vi "STAGE+mono+counter_edit12.vi"() -> ()   [LabVIEW 2017]
uses:
  Control 1.ctl
panel:
  out "XY Graph":cluster{dbl[], dbl[]}(graph)
  out "Slide":u8(slide) max=10 step=10 scale=0.0..10.0
  out "?":cluster{dbl[], "Y":T1}(graph)
  in  "?":enum32{"DELAY", "COUNTER", "MONO", "PLOT"}(tab)
  out "Final time [ps]":dbl
  out "Current time [ps]":dbl
  out "Initial time [ps]":dbl
  in  "Set this as t0":bool
  in  "Axis":i32=1
  in  "Motor ON":bool
  in  "Motor OFF":bool
  out "Current Position [mm]":dbl
  out "Final Position [mm]":dbl
  in  "Data Points":i32=100
  out "Current Point":i32
  in  "Step Size [um]":i32=10
  in  "Target [mm]":dbl format="%.3f"
  in  "Move":bool
  out "Initial position [mm]":dbl
  in  "GPIB address":string="23"
  in  "Count Mode":u16(ring) items=["A,B for Preset T", "A-B for Preset T", "A+B for Preset T", "A for Preset B"]
  in  "Trigger mode":u16(ring) items=["10 MHz"=0, "Input 2"=2, "Input T"=3]
  in  "Channel A Input":u16(ring)=1 items=["10 MHz", "Input 1"]
  in  "Channel B Input":u16(ring)=2 items=["Input 1"=1, "Input 2"=2]
  in  "Number of Measurements\n to take at one point/ Number of Periods":u16=1 min=1 max=2000 step=1
  in  "Time between measurements\n at one point (s)/Dwell Time":dbl=0.002 min=0.002 max=60.0 step=0.001
  in  "gate A mode (CW:0)":i16(slide) scale=0.0..2.0 scale format="%.2f"
  out "Counts":i32
  in  "Integrating time, 10^-7 sec":dbl=10000000.0
  out "Mono port":T2(ring)
  out "Time delay":u32=450000 min=1
  out "Serial":u32=12345
  in  "Step size":dbl=10.0 min=0.0
  in  "Scan to":i32=4000
  in  "Scan from":i32=2600
  out "Current wavelength":dbl
  out "Grt#":u8=1 min=1 max=3 step=1
  in  "?":bool
  out "Groove/mm":u32=1200
  out "Blaze (nm)":u32=300
  in  "Array":dbl[](array[numeric])
  out "Timeout 2":bool
  in  "?":bool
  out "Timeout":bool
  in  "Collect Data!":bool
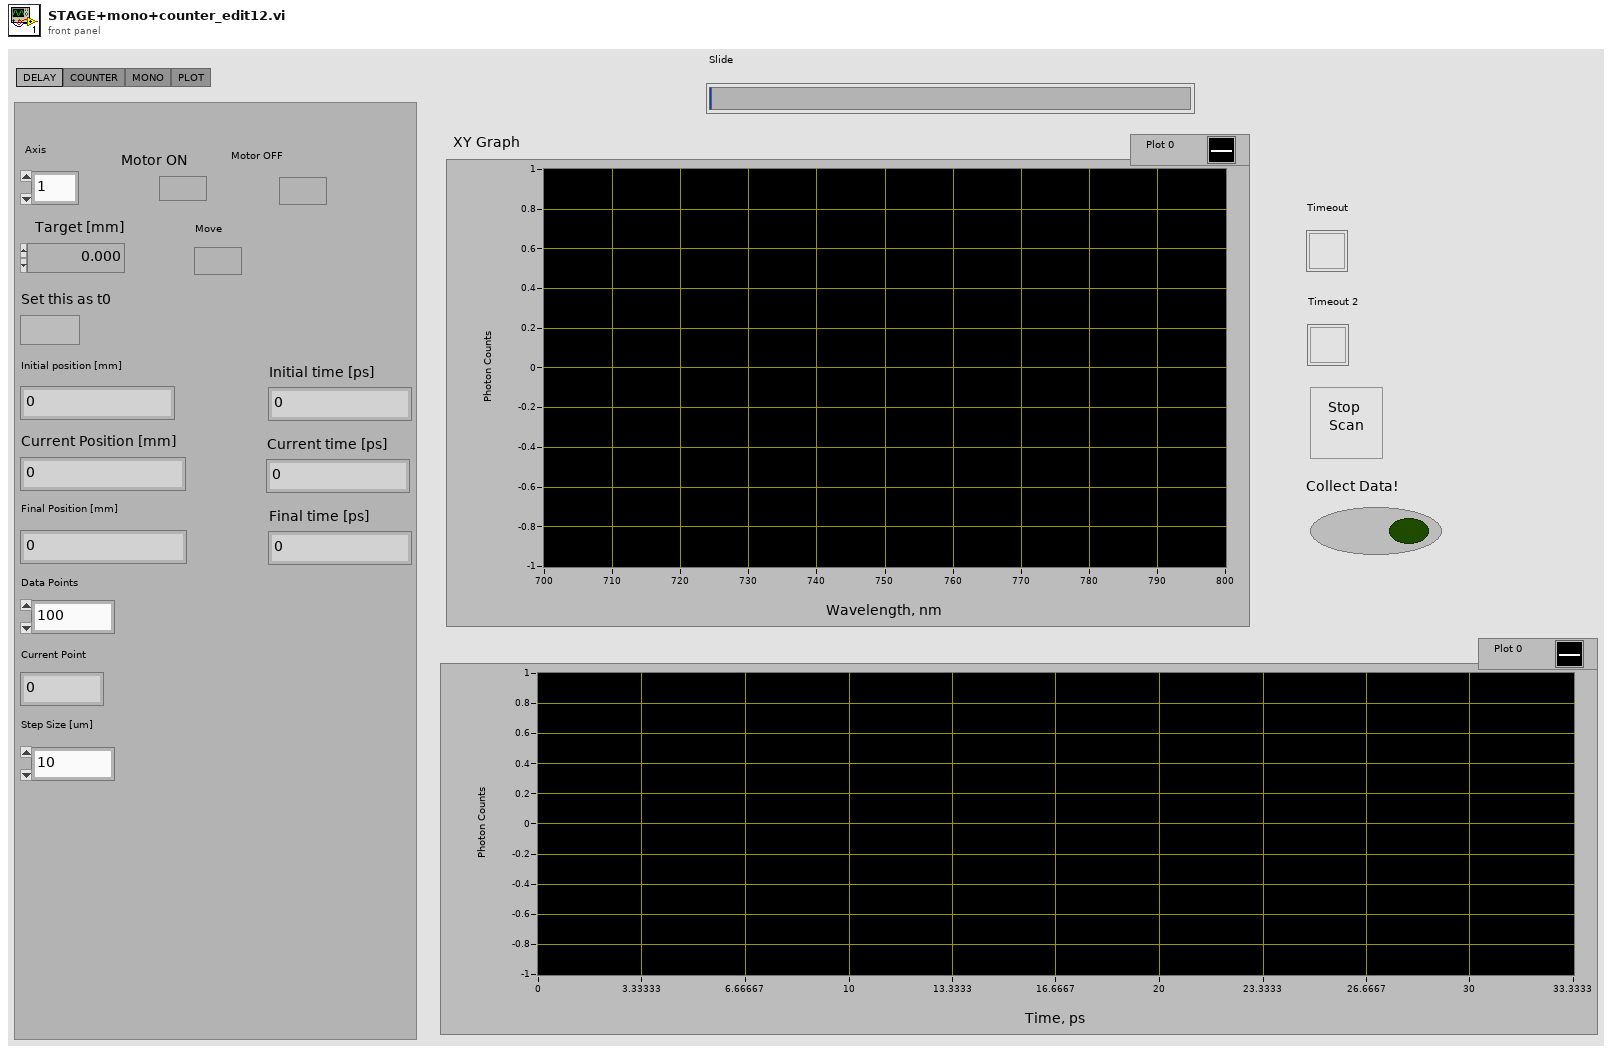
[diagram p1: front panel]
types:
  T1 = typedef "Control 1.ctl" = dbl[]
  T2 = enum8{"COM 1", "COM 2", "COM 3", "COM 4", "COM 5", "COM 6", "COM 7", "COM 8", "COM 9"}
  T3 = cluster{"input XON/XOFF":bool, "input HW Handshake":bool, "input alt HW HShk":bool, "output XON/XOFF":bool, "output HW Handshake":bool, "output alt HW HShk":bool, "XOFF byte":u8, "XON byte":u8, "parity error byte":u16}
  T4 = enum16{"no parity", "odd parity", "even parity", "mark parity", "space parity"}
  T5 = cluster{"Y[0]":dbl, "Y[1]":dbl, "Y[2]":dbl, "Y[3]":dbl, "Y[4]":dbl, "Y[5]":dbl, "Y[6]":dbl, "Y[7]":dbl, "Y[8]":dbl}
  T6 = typedef "NI_Matrix.lvlib/RealMatrix.ctl" = dbl[][]
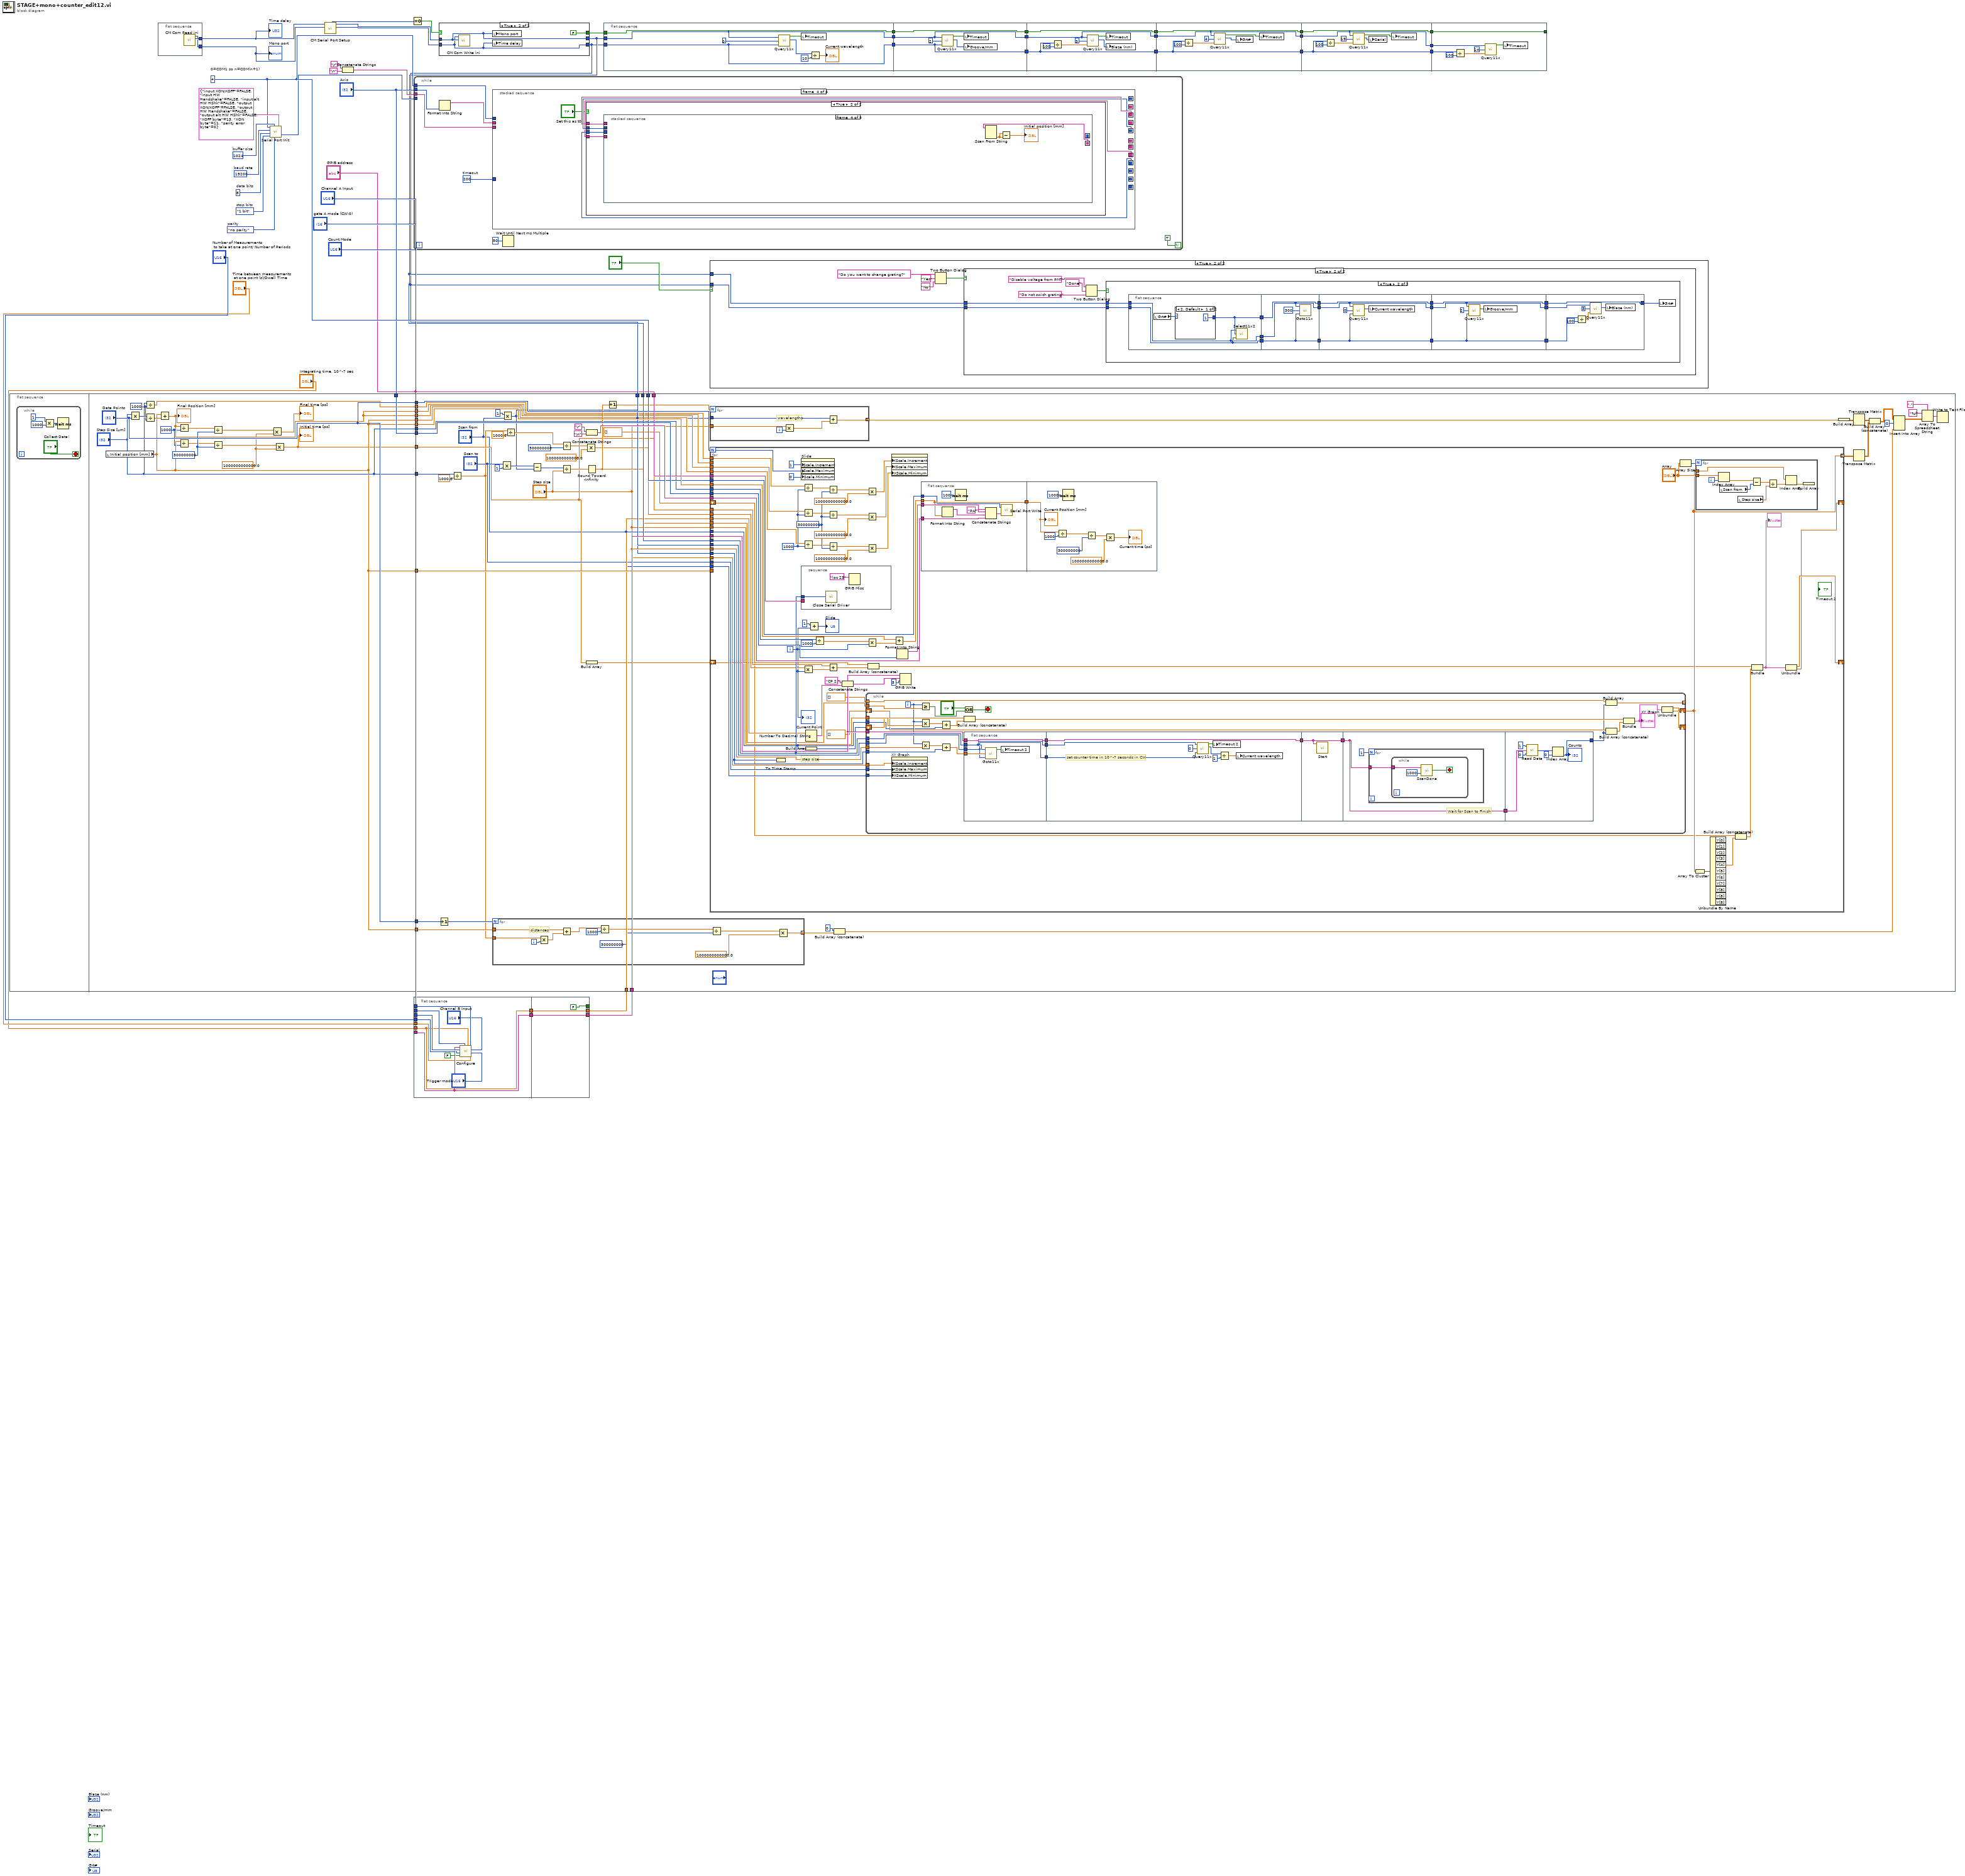
[diagram p0: block diagram]
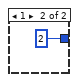
[diagram p5: hidden frame]
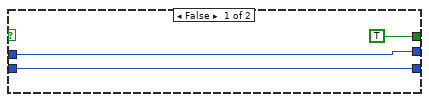
[diagram p6: hidden frame]
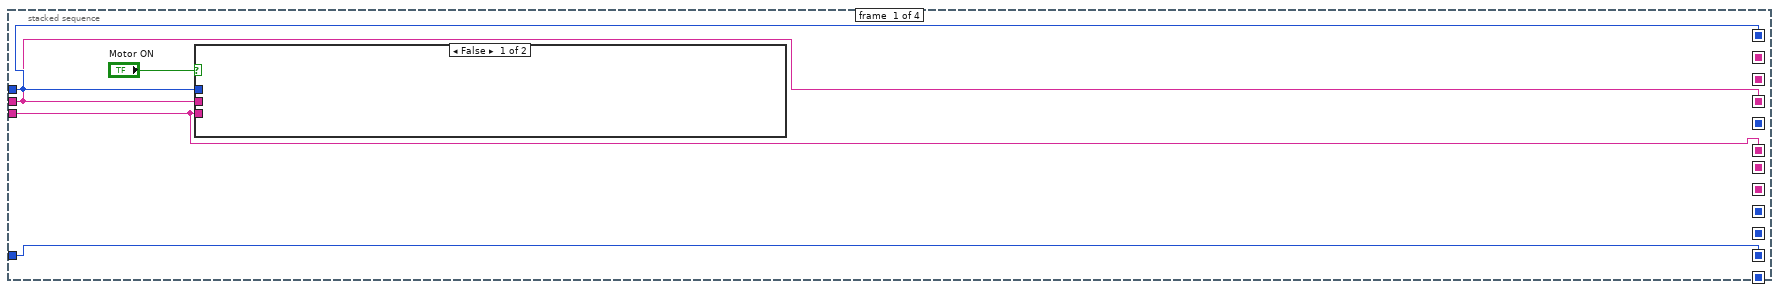
[diagram p7: hidden frame]
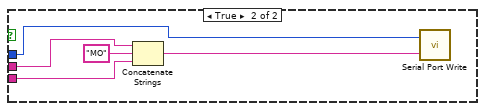
[diagram p8: hidden frame]
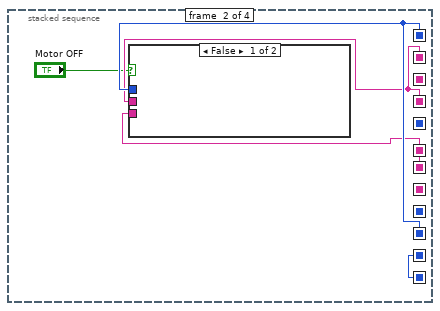
[diagram p9: hidden frame]
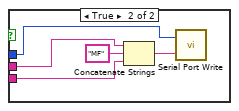
[diagram p10: hidden frame]
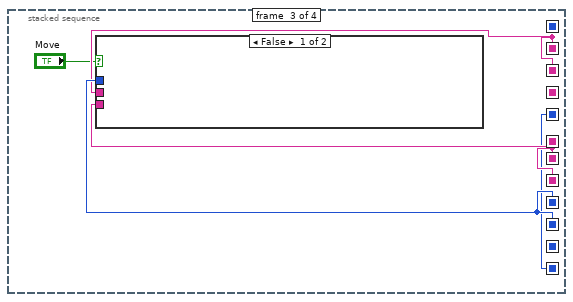
[diagram p11: hidden frame]
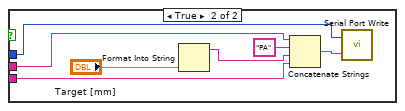
[diagram p12: hidden frame]
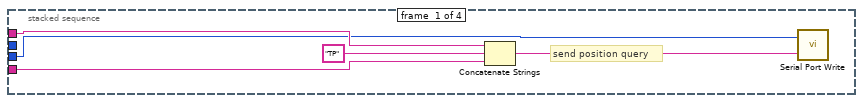
[diagram p14: hidden frame]
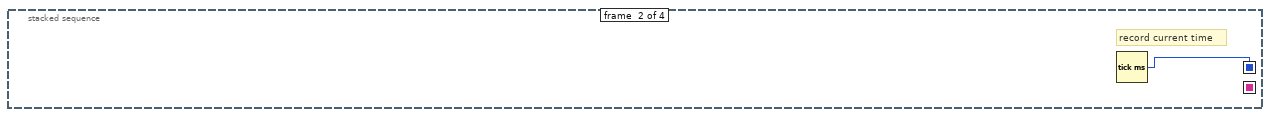
[diagram p15: hidden frame]
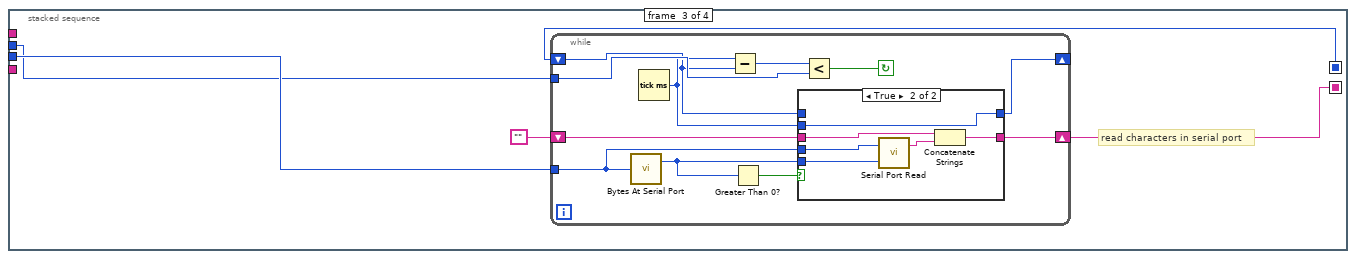
[diagram p16: hidden frame]
diagram:
  w55 = u32 19200  # baud rate
  w54 = u16 8  # data bits
  w53 = enum16{"1 bit", "1.5 bits", "2 bits"}."1 bit"  # stop bits
  w57 = T4."no parity"  # parity
  w52 = 4  # 0=COM1 so n=COM(n+1)
  w56 = u16 1024  # buffer size
  n1 = flat-sequence {
    tunnel: ["Data Points"] -> w61
    tunnel: "Axis" -> [w83]
    tunnel: [w75] -> w60
    tunnel: [w83] -> w59
    tunnel: ["Step Size [um]"] -> w12
    tunnel: [w75] -> w11
    tunnel: ["Step Size [um]"] -> w10
    tunnel: ["Data Points"] -> w9
    tunnel: [w75] -> w8
    tunnel: [w74] -> w7
    tunnel: [w75] -> w4
    tunnel: [w74] -> w3
    tunnel: [w77] -> w2
    tunnel: [w66] -> w1
    tunnel: w61 -> [w141]
    tunnel: w60 -> [w140]
    tunnel: w59 -> [w139]
    tunnel: w52 -> [w135]
    tunnel: w16 -> [w134]
    tunnel: w15 -> [w133]
    tunnel: w14 -> [w132]
    tunnel: "GPIB address" -> [w131]
    tunnel: w12 -> [w118]
    tunnel: w11 -> [w116]
    tunnel: w10 -> [w115]
    tunnel: w9 -> [w113]
    tunnel: w8 -> [w106]
    tunnel: w7 -> [w105]
    tunnel: w6 -> [w104]
    tunnel: w4 -> [w102]
    tunnel: w3 -> [w101]
    tunnel: w2 -> [w100]
    tunnel: w1 -> [w96]
    frame #0 {
      n2 = while {
        stop <- "Collect Data!" stop-if-true
        n3 = Multiply(x=1, y=1000) -> (x*y=w65:i32)
        n4 = Wait (ms)(milliseconds to wait=w65) -> ()  [unwired: 1 out]
      }
    }
    frame #1 {
      w67 = 1000000000000.0
      w73 = 1000
      w76 = 300000000
      w78 = 1000
      n5 = local read "Initial position [mm]"() -> (w75:dbl)
      n6 = Multiply(x="Step Size [um]", y="Data Points") -> (x*y=w82:i32)
      n7 = Divide(x="Step Size [um]", y=w78) -> (x/y=w77:dbl)
      n8 = Divide(x=w82, y=w78) -> (x/y=w81:dbl)
      n9 = Add(x=w75, y=w81) -> (x+y=w74:dbl)
      "Final Position [mm]" <- w74
      n10 = Divide(x=w74, y=w73) -> (x/y=w72:dbl)
      n11 = Divide(x=w75, y=w73) -> (x/y=w71:dbl)
      n12 = Divide(x=w72, y=w76) -> (x/y=w69:dbl)
      n13 = Divide(x=w71, y=w76) -> (x/y=w70:dbl)
      n14 = Multiply(x=w69, y=w67) -> (x*y=→"Final time [ps]":dbl)
      n15 = Multiply(x=w70, y=w67) -> (x*y=w66:dbl)
      "Initial time [ps]" <- w66
    }
    frame #2 {
      n16 = Increment(x=w113) -> (x+1=w114:i32)
      n17 = Divide(x=w118, y=1000.0) -> (x/y=w90:dbl)
      n18 = for {
        N: w114 -> [_]
        tunnel: w90 -> [w152]
        tunnel: w116 -> [w150]
        tunnel: [w143] -> w112 mode=indexing
        i -> [w151]
        # "distances"
        n19 = Multiply(x=w152, y=w151) -> (x*y=w149:dbl)
        n20 = Add(x=w150, y=w149) -> (x+y=w148:dbl)
        n21 = Divide(x=w148, y=1000) -> (x/y=w142:dbl)
        n22 = Divide(x=w142, y=300000000) -> (x/y=w145:dbl)
        n23 = Multiply(x=w145, y=1000000000000.0) -> (x*y=w143:dbl)
      }
      n24 = Multiply(x="Scan to", y=1) -> (x*y=w97:i32)
      n25 = Multiply(x=1, y="Scan from") -> (x*y=w86:i32)
      n26 = Divide(x=w90, y=1000.0) -> (x/y=w91:dbl)
      n27 = Subtract(x=w97, y=w86) -> (x-y=w126:i32)
      n28 = Divide(x=w91, y=300000000) -> (x/y=w93:dbl)
      n29 = Divide(x=w126, y="Step size") -> (x/y=w125:dbl)
      n30 = Multiply(x=w93, y=1000000000000.0) -> (x*y=w89:dbl)
      n31 = Concatenate Strings("\r", "\n") -> (w136:string)
      n32 = Round Toward -Infinity(1:w125) -> (0:w124:dbl)
      n33 = Build Array(w96) -> (w98:dbl[])
      n34 = Increment(x=w124) -> (x+1=w85:dbl)
      n35 = for {
        N: w85 -> [_]
        tunnel: "Step size" -> [w157]
        tunnel: w86 -> [w155]
        tunnel: [w153] -> w84 mode=indexing
        i -> [w156]
        # "wavelengths"
        n36 = Multiply(x=w157, y=w156) -> (x*y=w154:dbl)
        n37 = Add(x=w155, y=w154) -> (x+y=w153:dbl)
      }
      n38 = for {
        N: w141 -> [w193]
        tunnel: w140 -> [w227]
        tunnel: w115 -> [w223]
        tunnel: w139 -> [w220]
        tunnel: w136 -> [w217]
        tunnel: w135 -> [w218]
        tunnel: w134 -> [w216]
        tunnel: w133 -> [w213]
        tunnel: w132 -> [w215]
        tunnel: w131 -> [w214]
        tunnel: [w160] -> w121 mode=indexing
        tunnel: w86 -> [w208]
        tunnel: "Step size" -> [w207]
        tunnel: w124 -> [w206]
        tunnel: w106 -> [_]
        tunnel: w105 -> [_]
        tunnel: w104 -> [w204]
        tunnel: "Scan to" -> [w203]
        tunnel: "Scan from" -> [w202]
        tunnel: "Step size" -> [w164]
        tunnel: w102 -> [w188]
        tunnel: w101 -> [w186]
        tunnel: w100 -> [w189]
        tunnel: w89 -> [w173]
        shift-right: [w200] -> _
        shift-left: w98 -> [w167]
        shift-right: [w197] -> _
        shift-left: T1 [] ("Y") -> [w158]
        tunnel: w96 -> [w196]
        tunnel: "Scan from" -> [w165]
        tunnel: "Step size" -> [w166]
        i -> [w172]
        w187 = 1000
        w190 = 300000000
        # "step size"
        n39 = To Time Stamp(1:w208) -> ()  [unwired: 1 out]
        n40 = property on="Slide" class="Slide (strict)"("Scale.Increment"=1, "Scale.Maximum"=w193, "Scale.Minimum"=0) -> ()  [unwired: 2 in, 2 out]
        n41 = stacked-sequence {
          tunnel: w213 -> [w299]
          tunnel: w214 -> [_]
          frame #0 {
            n42 = call <vilib>:"Close Serial Driver.vi"("port number"=w299) -> ()  [unwired: 1 out]
            n43 = GPIB Misc(0:"loc 23" ("command string")) -> ()  [unwired: 1 in, 3 out]
          }
        }
        n44 = Divide(x=w189, y=w187) -> (x/y=w185:dbl)
        n45 = Divide(x=w186, y=w187) -> (x/y=w183:dbl)
        n46 = Divide(x=w188, y=w187) -> (x/y=w184:dbl)
        n47 = Multiply(x=w173, y=w172) -> (x*y=w201:dbl)
        n48 = Number To Decimal String(number=w204) -> (decimal integer string=w211:string)  [unwired: 1 in]
        n49 = Build Array(w165) -> (w169:i32[])
        n50 = Add(x=1, y=w172) -> (x+y=→"Slide":i32)
        n51 = Divide(x=w223, y=1000) -> (x/y=w222:dbl)
        n52 = Divide(x=w185, y=w190) -> (x/y=w179:dbl)
        n53 = Divide(x=w183, y=w190) -> (x/y=w175:dbl)
        n54 = Divide(x=w184, y=w190) -> (x/y=w177:dbl)
        n55 = Add(x=w196, y=w201) -> (x+y=w195:dbl)
        n56 = Concatenate Strings("CP 2,", w211) -> (w209:string)
        n57 = while {
          tunnel: w213 -> [w270]
          tunnel: w215 -> [w269]
          tunnel: w216 -> [w265]
          tunnel: w208 -> [w257]
          tunnel: w207 -> [w256]
          tunnel: w206 -> [w255]
          tunnel: w203 -> [w242]
          tunnel: w202 -> [w241]
          tunnel: w164 -> [w240]
          tunnel: w166 -> [w253]
          shift-right: [w248] -> w160
          shift-left: dbl[] [] ("Y") -> [w247]
          shift-right: [w237] -> _
          shift-left: w169 -> [w251]
          tunnel: w165 -> [w245]
          tunnel: dbl[] [] ("Y") -> [w238] mode=indexing
          tunnel: [w239] -> _ mode=indexing
          i -> [w254]
          stop <- w268 stop-if-true
          n58 = property on="XY Graph" class="XYGraph (strict)"("XScale.Increment"=w240, "XScale.Maximum"=w242, "XScale.Minimum"=w241) -> ()  [unwired: 2 in, 2 out]
          n59 = Greater Or Equal?(x=w254, y=w255) -> (x >= y?=w266:bool)
          n60 = Multiply(x=w254, y=w253) -> (x*y=w252:dbl)
          n61 = Multiply(x=w254, y=w256) -> (x*y=w271:dbl)
          n62 = Add(x=w252, y=w245) -> (x+y=w250:dbl)
          n63 = Add(x=w271, y=w257) -> (x+y=w258:dbl)
          n64 = Or(x="?", y=w266) -> (x .or. y?=w268:bool)
          n65 = Build Array (concatenate)(w251, w250) -> (w249:dbl[])
          n66 = flat-sequence {
            tunnel: w258 -> [w276]
            tunnel: w270 -> [w275]
            tunnel: [w275] -> w264
            tunnel: w269 -> [w274]
            tunnel: [w274] -> w263
            tunnel: w265 -> [w272]
            tunnel: [w272] -> w262
            tunnel: w264 -> [w283]
            tunnel: w263 -> [w282]
            tunnel: w262 -> [w280]
            tunnel: [w280] -> w261
            tunnel: w261 -> [w285]
            tunnel: [w285] -> w260
            tunnel: w260 -> [w286]
            tunnel: [w286] -> w259
            tunnel: w259 -> [w293]
            tunnel: [w292] -> w244
            frame #0 {
              n67 = call "Goto11x.vi"("time delay"=w274, "WAVELENGTH"=w276, "port number"=w275) -> ("timeout"=w273:bool)  [unwired: 2 out]
              n68 = local write "Timeout 2"(w273) -> ()
            }
            frame #1 {
              # "set counter time in 10^-7 seconds in CW"
              n69 = call "Query11x.vi"("port number"=w283, "QUERY"=0, "time delay"=w282) -> ("timeout"=w281:bool, "STATUS MESSAGE"=w279:u16)  [unwired: 2 out]
              n70 = local write "Timeout 2"(w281) -> ()
              n71 = Divide(x=w279, y=1) -> (x/y=w278:dbl)
              n72 = local write "Current wavelength"(w278) -> ()
            }
            frame #2 {
              n73 = call "Start.vi"("GPIB Address"=w285) -> ()  [unwired: 9 in]
            }
            frame #3 {
              # "Wait for Scan to Finish"
              n74 = for {
                N: 1 -> [_]
                tunnel: w286 -> [w288]
                n75 = while {
                  tunnel: w288 -> [w289]
                  stop <- w291 stop-if-true
                  n76 = call "ScanDone.vi"("Wait (ms)"=1000, "GPIB Address"=w289) -> ("Scan Finished?"=w291:bool)
                }
              }
            }
            frame #4 {
              n77 = call "Read Data.vi"("Channel Number"=0, "GPIB Address"=w293, "Number of Datapoints"=1) -> ("Data"=w294:i32[])
              n78 = Index Array(array=w294, index=0) -> (element=w292:i32)
              "Counts" <- w292
            }
          }
          n79 = Build Array(w238, w244) -> (w239:dbl[])
          n80 = Build Array (concatenate)(w247, w244) -> (w246:dbl[])
          n81 = Bundle(w249, w246) -> (w243:cluster{dbl[], dbl[]})  [unwired: 1 in]
          "XY Graph" <- w243
          n82 = Unbundle(w243) -> (w237:dbl[], w248:dbl[])
        }
        n83 = Multiply(x=w179, y=1000000000000.0) -> (x*y=w178:dbl)
        n84 = Multiply(x=w175, y=1000000000000.0) -> (x*y=w174:dbl)
        n85 = Multiply(x=w177, y=1000000000000.0) -> (x*y=w176:dbl)
        n86 = Multiply(x=w222, y=w172) -> (x*y=w226:dbl)
        n87 = Build Array (concatenate)(w167, w195) -> (w159:dbl[])
        n88 = property class="XYGraph (strict)"("XScale.Increment"=w178, "XScale.Maximum"=w174, "XScale.Minimum"=w176) -> ()  [unwired: 2 in, 2 out]
        n89 = Add(x=w227, y=w226) -> (x+y=w225:dbl)
        n90 = Format Into String(w220) -> (resulting string=w219:string)  [unwired: 3 in, 1 out]
        n91 = GPIB Write(0:w216, 1:w209, 2:i16 5 ("mode (0)")) -> ()  [unwired: 2 in, 2 out]
        n92 = flat-sequence {
          tunnel: w225 -> [w302]
          tunnel: [w302] -> w221
          tunnel: w217 -> [w304]
          tunnel: w219 -> [w303]
          tunnel: w218 -> [w300]
          tunnel: w221 -> [w313]
          frame #0 {
            n93 = Format Into String(w302) -> (resulting string=w301:string)  [unwired: 3 in, 1 out]
            n94 = Wait (ms)(milliseconds to wait=u32 100) -> ()  [unwired: 1 out]
            n95 = Concatenate Strings(w303, "PA" ("Substring"), w301, w304) -> (w306:string)
            n96 = call <vilib>:"Serial Port Write.vi"("string to write"=w306, "port number"=w300) -> ()  [unwired: 1 out]
          }
          frame #1 {
            n97 = Divide(x=w313, y=1000) -> (x/y=w311:dbl)
            n98 = Wait (ms)(milliseconds to wait=u32 1000) -> ()  [unwired: 1 out]
            n99 = Divide(x=w311, y=300000000) -> (x/y=w310:dbl)
            n100 = Multiply(x=w310, y=1000000000000.0) -> (x*y=→"Current time [ps]":dbl)
            "Current Position [mm]" <- w313
          }
        }
        n101 = Array Size(array="Array") -> (size(s)=w162:i32)
        n102 = Array To Cluster(array=w160) -> (cluster=w205:T5)
        n103 = for {
          N: w162 -> [_]
          tunnel: "Array" -> [w236]
          tunnel: w160 -> [w230]
          i -> [w235]
          n104 = Index Array(array=w236, index=w235) -> (element=w234:dbl)
          n105 = local read "Scan from"() -> (w233:i32)
          n106 = local read "Step size"() -> (w231:dbl)
          n107 = Subtract(x=w234, y=w233) -> (x-y=w232:dbl)
          n108 = Divide(x=w232, y=w231) -> (x/y=w229:dbl)
          n109 = Index Array(array=w230, index=w229) -> (element=w228:dbl)
          n110 = Build Array(w228) -> ()  [unwired: 1 out]
        }
        n111 = Unbundle By Name(w205) -> ("Y[4]"=w199:dbl)  [unwired: 10 out]
        n112 = Build Array (concatenate)(w158, w199) -> (w198:T1)
        n113 = Bundle(w159, "Y"=w198) -> (w194:cluster{dbl[], "Y":T1})  [unwired: 1 in]
        "?" <- w194
        n114 = Unbundle(w194) -> (w200:dbl[], "Y"=w197:T1)
        "Current Point" <- w172
      }
      n115 = Build Array (concatenate)(0, w112) -> (w109:dbl[])
      n116 = Build Array(w84) -> (w122:dbl[][])
      n117 = Transpose Matrix(1:w122) -> (0:w120:dbl[][])
      n118 = Transpose Matrix(1:w121) -> (0:w119:dbl[][])
      n119 = Build Array (concatenate)(w120, w119) -> (w108:T6)
      n120 = Insert Into Array(array=w108, index (row)=0, new element=w109) -> (w107:T6)  [unwired: 1 in]
      n121 = Array To Spreadsheet String(delimiter (Tab)=",", array=w107, 3:"%f" ("format string")) -> (spreadsheet string=w123:string)
      n122 = Write to Text File(text=w123) -> ()  [unwired: 3 in, 3 out]
    }
  }
  n123 = flat-sequence {
    tunnel: [w317] -> w30
    tunnel: [w316] -> w29
    frame #0 {
      n124 = call "CM Com Read ini.vi"() -> ("Mono port"=w316:T2, "time delay1"=w317:u32)  [unwired: 7 in]
    }
  }
  n125 = call <vilib>:"Serial Port Init.vi"("flow control etc."=T3 {"input XON/XOFF"=FALSE, "input HW Handshake"=FALSE, "input alt HW HShk"=FALSE, "output XON/XOFF"=FALSE, "output HW Handshake"=FALSE, "output alt HW HShk"=FALSE, "XOFF byte"=13, "XON byte"=11, "parity error byte"=0}, "parity"=w57, "buffer size"=w56, "stop bits"=w53, "data bits"=w54, "baud rate"=w55, "port number"=w52) -> ("error code"=w51:i32)
  n126 = call "CM Serial Port Setup.vi"("COM port"=w29, "time delay"=w30) -> ("time delay1"=w25:u32, "DK port Out"=w26:T2, "error code"=w28:i32)  [unwired: 7 in]
  n127 = Concatenate Strings("\r", "\n") -> (w47:string)
  n128 = Equal To 0?(x=w28) -> (x = 0?=w27:bool)
  n129 = while {
    tunnel: w52 -> [w320]
    tunnel: w47 -> [w321]
    tunnel: w51 -> [_]
    tunnel: "Axis" -> [w318]
    stop <- TRUE continue-if-true
    w319 = u32 200  # timeout
    n130 = Format Into String(w318) -> (resulting string=w322:string)  [unwired: 3 in, 1 out]
    n131 = stacked-sequence {
      seq-local: [w327 _ _ _] -> [_ w338 _ _]
      seq-local: [w326 _ _ _] -> [_ w337 _ _]
      seq-local: [w328 _ _ _] -> [_ w339 _ _]
      seq-local: [w325 _ _ _] -> [_ w335 _ _]
      seq-local: [_ w338 _ _] -> [_ _ w348 _]
      seq-local: [_ w337 _ _] -> [_ _ w347 _]
      seq-local: [_ w339 _ _] -> [_ _ w349 _]
      seq-local: [_ w335 _ _] -> [_ _ w345 _]
      seq-local: [_ _ w348 _] -> [_ _ _ w361]
      seq-local: [_ _ w347 _] -> [_ _ _ w358]
      seq-local: [_ _ w349 _] -> [_ _ _ w360]
      seq-local: [_ _ w345 _] -> [_ _ _ w359]
      tunnel: w322 -> [w327 _ _ _]
      tunnel: w321 -> [w326 _ _ _]
      tunnel: w320 -> [w328 _ _ _]
      tunnel: w319 -> [w325 _ _ _]
      frame #0 {
        n132 = case shown="False" "Motor ON" {
          tunnel: w328 -> [_ w334]
          tunnel: w327 -> [_ w331]
          tunnel: w326 -> [_ w330]
          frame False {
          }
          frame True {
            n133 = Concatenate Strings(w331, "MO" ("Substring"), w330) -> (w332:string)
            n134 = call <vilib>:"Serial Port Write.vi"("string to write"=w332, "port number"=w334) -> ()  [unwired: 1 out]
          }
        }
      }
      frame #1 {
        n135 = case shown="False" "Motor OFF" {
          tunnel: w339 -> [_ w344]
          tunnel: w338 -> [_ w341]
          tunnel: w337 -> [_ w340]
          frame False {
          }
          frame True {
            n136 = Concatenate Strings(w341, "MF" ("Substring"), w340) -> (w342:string)
            n137 = call <vilib>:"Serial Port Write.vi"("string to write"=w342, "port number"=w344) -> ()  [unwired: 1 out]
          }
        }
      }
      frame #2 {
        n138 = case shown="False" "Move" {
          tunnel: w349 -> [_ w356]
          tunnel: w348 -> [_ w353]
          tunnel: w347 -> [_ w352]
          frame False {
          }
          frame True {
            n139 = Format Into String("Target [mm]") -> (resulting string=w350:string)  [unwired: 3 in, 1 out]
            n140 = Concatenate Strings(w353, "PA" ("Substring"), w350, w352) -> (w354:string)
            n141 = call <vilib>:"Serial Port Write.vi"("string to write"=w354, "port number"=w356) -> ()  [unwired: 1 out]
          }
        }
      }
      frame #3 {
        n142 = case shown="True" "Set this as t0" {
          tunnel: w361 -> [_ w365]
          tunnel: w360 -> [_ w364]
          tunnel: w359 -> [_ w363]
          tunnel: w358 -> [_ w362]
          frame False {
          }
          frame True {
            n143 = stacked-sequence {
              seq-local: [_ w371 _ _] -> [_ _ w373 _]
              seq-local: [_ _ w372 _] -> [_ _ _ w398]
              tunnel: w365 -> [w368 _ _ _]
              tunnel: w364 -> [w367 _ w376 _]
              tunnel: w363 -> [_ _ w374 _]
              tunnel: w362 -> [w366 _ _ _]
              frame #0 {
                # "send position query"
                n144 = Concatenate Strings(w368, "TP" ("Substring"), w366) -> (w369:string)
                n145 = call <vilib>:"Serial Port Write.vi"("string to write"=w369, "port number"=w367) -> ()  [unwired: 1 out]
              }
              frame #1 {
                # "record current time"
                n146 = Tick Count (ms)() -> (millisecond timer value=w371:u32)
              }
              frame #2 {
                # "read characters in serial port"
                n147 = while {
                  shift-left: w373 -> [w377]
                  shift-right: [w378] -> _
                  tunnel: w374 -> [w381]
                  shift-left: "" -> [w384]
                  shift-right: [w383] -> w372
                  tunnel: w376 -> [w385]
                  stop <- w380 continue-if-true
                  n148 = call <vilib>:"Bytes At Serial Port.vi"("port number"=w385) -> ("byte count"=w386:u32)  [unwired: 1 out]
                  n149 = Tick Count (ms)() -> (millisecond timer value=w379:u32)
                  n150 = Subtract(x=w379, y=w377) -> (x-y=w382:u32)
                  n151 = Greater Than 0?(x=w386) -> (x > 0?=w387:bool)
                  n152 = case shown="True" w387 {
                    tunnel: w386 -> [_ w395]
                    tunnel: w385 -> [_ w394]
                    tunnel: w384 -> [w389 w392]
                    tunnel: [w389 w391] -> w383
                    tunnel: [w388 w390] -> w378
                    tunnel: w379 -> [_ w390]
                    tunnel: w377 -> [w388 _]
                    frame False {
                    }
                    frame True {
                      n153 = call <vilib>:"Serial Port Read.vi"("requested byte count"=w395, "port number"=w394) -> ("string read"=w393:string)  [unwired: 1 out]
                      n154 = Concatenate Strings(w392, w393) -> (w391:string)
                    }
                  }
                  n155 = Less?(x=w382, y=w381) -> (x < y?=w380:bool)
                }
              }
              frame #3 {
                n156 = Scan From String(input string=w398) -> (output 1=w396:dbl)  [unwired: 4 in, 3 out]
                n157 = Subtract(x=w396, y=w396) -> (x-y=→"Initial position [mm]":dbl)
              }
            }
          }
        }
      }
    }
    n158 = Wait Until Next ms Multiple(millisecond multiple=u32 50) -> ()  [unwired: 1 out]
  }
  n159 = flat-sequence {
    tunnel: "GPIB address" -> [w406]
    tunnel: [w406] -> w31
    tunnel: "Count Mode" -> [w407]
    tunnel: "Number of Measurements\n to take at one point/ Number of Periods" -> [w404]
    tunnel: "Time between measurements\n at one point (s)/Dwell Time" -> [w403]
    tunnel: "Channel A Input" -> [w408]
    tunnel: "gate A mode (CW:0)" -> [w400]
    tunnel: "Integrating time, 10^-7 sec" -> [w399]
    tunnel: [w399] -> w5
    tunnel: w31 -> [w410]
    tunnel: [w410] -> w16
    tunnel: [FALSE] -> _
    tunnel: [w409] -> w6
    tunnel: w5 -> [w409]
    frame #0 {
      n160 = call "Configure.vi"("Dwell Time (s)"=w403, "Channel T Input"="Trigger mode", "Channel B Input"="Channel B Input", "Channel A Input"=w408, "Integrating time, 10^-7 sec"=w399, "gate mode (CW:0)"=w400, "Scan End Mode"=FALSE, "Number of Periods"=w404, "Count Mode"=w407, "GPIB Address"=w406) -> ()
    }
    frame #1 {
    }
  }
  n161 = case shown="True" w27 {
    tunnel: w26 -> [w414 w417]
    tunnel: w25 -> [w413 w416]
    tunnel: [w414 w417] -> w15
    tunnel: [w413 w416] -> w14
    tunnel: [TRUE FALSE] -> w24
    frame False {
    }
    frame True {
      n162 = call "CM Com Write ini.vi"("time delay1"=w417, "Mono port"=w416) -> ()  [unwired: 7 in]
      n163 = local write "Mono port"(w417) -> ()
      n164 = local write "Time delay"(w416) -> ()
    }
  }
  n165 = flat-sequence {
    tunnel: w14 -> [w423]
    tunnel: [w423] -> w46
    tunnel: w15 -> [w425]
    tunnel: [w425] -> w45
    tunnel: w24 -> [w421]
    tunnel: [w421] -> w44
    tunnel: w46 -> [w428]
    tunnel: [w428] -> w43
    tunnel: w45 -> [w430]
    tunnel: [w430] -> w42
    tunnel: w44 -> [w426]
    tunnel: [w426] -> w41
    tunnel: w43 -> [w438]
    tunnel: [w438] -> w40
    tunnel: w42 -> [w435]
    tunnel: [w435] -> w39
    tunnel: w41 -> [w432]
    tunnel: [w432] -> w38
    tunnel: w40 -> [w446]
    tunnel: [w446] -> w37
    tunnel: w39 -> [w443]
    tunnel: [w443] -> w36
    tunnel: w38 -> [w440]
    tunnel: [w440] -> w35
    tunnel: w37 -> [w454]
    tunnel: [w454] -> w34
    tunnel: w36 -> [w451]
    tunnel: [w451] -> w33
    tunnel: w35 -> [w448]
    tunnel: [w448] -> w32
    tunnel: w34 -> [w461]
    tunnel: w33 -> [w458]
    tunnel: [w456] -> _
    tunnel: w32 -> [w456]
    frame #0 {
      n166 = call "Query11x.vi"("port number"=w425, "QUERY"=u16 0, "time delay"=w423) -> ("timeout"=w422:bool, "STATUS MESSAGE"=w420:u16)  [unwired: 2 out]
      n167 = local write "Timeout"(w422) -> ()
      n168 = Divide(x=w420, y=10 ("Numeric")) -> (x/y=→"Current wavelength":dbl)
    }
    frame #1 {
      n169 = call "Query11x.vi"("port number"=w430, "QUERY"=u16 2, "time delay"=w428) -> ("timeout"=w427:bool, "STATUS MESSAGE"=w429:u16)  [unwired: 2 out]
      n170 = local write "Timeout"(w427) -> ()
      n171 = local write "Groove/mm"(w429) -> ()
    }
    frame #2 {
      n172 = Divide(x=w438, y=i16 100 ("device (1)")) -> (x/y=w436:dbl)
      n173 = call "Query11x.vi"("port number"=w435, "QUERY"=u16 3, "time delay"=w436) -> ("timeout"=w433:bool, "STATUS MESSAGE"=w434:u16)  [unwired: 2 out]
      n174 = local write "Timeout"(w433) -> ()
      n175 = local write "Blaze (nm)"(w434) -> ()
    }
    frame #3 {
      n176 = Divide(x=w446, y=i16 100 ("device (1)")) -> (x/y=w444:dbl)
      n177 = call "Query11x.vi"("port number"=w443, "QUERY"=u16 4, "time delay"=w444) -> ("timeout"=w441:bool, "STATUS MESSAGE"=w442:u16)  [unwired: 2 out]
      n178 = local write "Grt#"(w442) -> ()
      n179 = local write "Timeout"(w441) -> ()
    }
    frame #4 {
      n180 = Divide(x=w454, y=i16 100 ("device (1)")) -> (x/y=w452:dbl)
      n181 = call "Query11x.vi"("port number"=w451, "QUERY"=u16 19, "time delay"=w452) -> ("timeout"=w449:bool, "STATUS MESSAGE"=w450:u16)  [unwired: 2 out]
      n182 = local write "Serial"(w450) -> ()
      n183 = local write "Timeout"(w449) -> ()
    }
    frame #5 {
      n184 = Divide(x=w461, y=i16 100 ("device (1)")) -> (x/y=w459:dbl)
      n185 = call "Query11x.vi"("port number"=w458, "QUERY"=u16 14, "time delay"=w459) -> ("timeout"=w457:bool)  [unwired: 3 out]
      n186 = local write "Timeout"(w457) -> ()
    }
  }
  n187 = case shown="True" "?" {
    tunnel: w14 -> [_ w464]
    tunnel: w15 -> [_ w463]
    frame False {
    }
    frame True {
      n188 = Two Button Dialog(message="Do you want to change grating?", 1:"No" ("F button name (\"Cancel\")"), 2:"Yes" ("T button name (\"OK\")")) -> (T button?=w465:bool)
      n189 = case shown="True" w465 {
        tunnel: w464 -> [_ w470]
        tunnel: w463 -> [_ w469]
        frame False {
        }
        frame True {
          n190 = Two Button Dialog(message="Disable voltage from PMT", 1:"Do not swich grating" ("F button name (\"Cancel\")"), 2:"Done" ("T button name (\"OK\")")) -> (T button?=w471:bool)
          n191 = case shown="True" w471 {
            tunnel: w470 -> [_ w489]
            tunnel: w469 -> [_ w488]
            frame False {
            }
            frame True {
              n192 = flat-sequence {
                tunnel: w489 -> [w493]
                tunnel: [w493] -> w486
                tunnel: w488 -> [w492]
                tunnel: [w492] -> w485
                tunnel: [w490] -> w484
                tunnel: w486 -> [w497]
                tunnel: [w497] -> w483
                tunnel: w485 -> [w498]
                tunnel: [w498] -> w482
                tunnel: w484 -> [w496]
                tunnel: [w496] -> w481
                tunnel: w483 -> [w504]
                tunnel: [w504] -> w480
                tunnel: w482 -> [w503]
                tunnel: [w503] -> w479
                tunnel: w481 -> [w501]
                tunnel: [w501] -> w478
                tunnel: w480 -> [w507]
                tunnel: [w507] -> w477
                tunnel: w479 -> [w508]
                tunnel: [w508] -> w476
                tunnel: w478 -> [w505]
                tunnel: [w505] -> w475
                tunnel: w477 -> [w512]
                tunnel: w476 -> [w513]
                tunnel: [w510] -> w487
                tunnel: w475 -> [w510]
                frame #0 {
                  n193 = local read "Grt#"() -> (w491:u8)
                  n194 = case shown="2, Default" w491 {
                    tunnel: [1 2] -> w490
                    frame 2, Default {
                    }
                    frame 1 {
                    }
                  }
                  n195 = call "Select11x2.vi"("time delay"=w493, "NEW GRT?"=w490, "port number"=w492) -> ()  [unwired: 3 out]
                }
                frame #1 {
                  n196 = call "Goto11x.vi"("time delay"=w497, "WAVELENGTH"=u16 300, "port number"=w498) -> ()  [unwired: 3 out]
                }
                frame #2 {
                  n197 = call "Query11x.vi"("port number"=w503, "QUERY"=u16 0, "time delay"=w504) -> ("STATUS MESSAGE"=w500:u16)  [unwired: 3 out]
                  n198 = local write "Current wavelength"(w500) -> ()
                }
                frame #3 {
                  n199 = call "Query11x.vi"("port number"=w508, "QUERY"=u16 2, "time delay"=w507) -> ("STATUS MESSAGE"=w506:u16)  [unwired: 3 out]
                  n200 = local write "Groove/mm"(w506) -> ()
                }
                frame #4 {
                  n201 = Divide(x=w512, y=i16 100 ("device (1)")) -> (x/y=w514:dbl)
                  n202 = call "Query11x.vi"("port number"=w513, "QUERY"=u16 3, "time delay"=w514) -> ("STATUS MESSAGE"=w511:u16)  [unwired: 3 out]
                  n203 = local write "Blaze (nm)"(w511) -> ()
                }
              }
              n204 = local write "Grt#"(w487) -> ()
            }
          }
        }
      }
    }
  }
  "Mono port" <- w29
  "Time delay" <- w30
